vi "FIFO Core U128 - DRAM.vi"(0 "input data":cluster{"high":u64, "low":u64}, 1 "reset":bool, 2 "fifo memory":refnum<k21>, 3 "fifo depth":u8(ring)=10 items=["4"=2, "8"=3, "16"=4, "32"=5, "64"=6, "128"=7, "256"=8, "512"=9, "1024"=10, "2048"=11, "4096"=12, "8192"=13, "16384"=14, "32768"=15, "65536"=16, "131072"=17, "262144"=18, "524288"=19, "1048576"=20, "2097152"=21, "4194304"=22, "8388608"=23, "16777216"=24, "33554432"=25, "67108864"=26, "134217728"=27, "268435456"=28, "536870912"=29, "1073741824"=30, "2147483648"=31, "4294967296"=32], 5 "arbiter configuration":T2={"write grant time (clocks)"=100, "read grant time (clocks)"=100}, 9 "input valid":bool, 12 "ready for output":bool=TRUE) -> (4 "output data":cluster{"high":u64, "low":u64}, 6 "state":T1, 10 "output valid":bool, 14 "ready for input":bool)   [LabVIEW 2011, in "FIFO.lvlib"]
uses:
  <instrlib>/RF-RIO/FIFO/FIFO/FPGA/FIFO.lvlib
  <instrlib>/RF-RIO/FIFO/FIFO/FPGA/Public/FIFO State.ctl
  <instrlib>/RF-RIO/Memory/1.0.0/FPGA/Public/Write Data (128-Bit).ctl
  <instrlib>/RF-RIO/Memory/1.0.0/FPGA/Public/U128.ctl
  <instrlib>/FlexRIO/Libraries/Memory/FPGA/Interface/Read Request.ctl
  <instrlib>/RF-RIO/Memory/1.0.0/FPGA/Private/Process (DRAM 128-Bit).vi
  <instrlib>/FlexRIO/Libraries/Memory/FPGA/Memory.lvlib
  <instrlib>/RF-RIO/Memory/1.0.0/FPGA/niRFRIO Memory 1.0.0 FPGA.lvlib
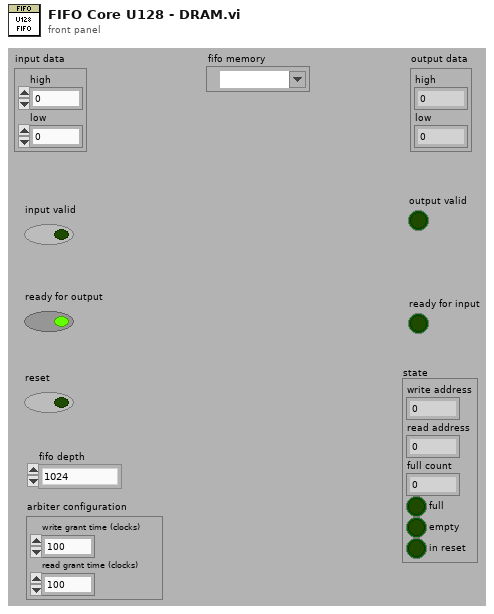
[diagram p1: front panel]
types:
  T1 = typedef "FIFO.lvlib/FIFO State.ctl" = cluster{"write address":u32, "read address":u32, "full count":u32, "full":bool, "empty":bool, "in reset":bool}
  T2 = cluster{"write grant time (clocks)":u16, "read grant time (clocks)":u16}
  T3 = typedef "Memory.lvlib/Read Request.ctl" = cluster{"address":u32, "valid":bool}
  T4 = typedef "FIFO.lvlib/niRFRIO Memory 1.0.0 FPGA.lvlib/Write Data (128-Bit).ctl" = cluster{"address":u32, "data":T5, "byte enables":u16, "valid":bool}
  T5 = typedef "FIFO.lvlib/niRFRIO Memory 1.0.0 FPGA.lvlib/U128.ctl" = cluster{"high":u64, "low":u64}
  T6 = typedef "FIFO.lvlib/FIFO State - 32-bit Address.ctl" = cluster{"write address":u32, "read address":u32, "full count":u32, "full":bool, "empty":bool}
  T7 = typedef "FIFO.lvlib/niRFRIO Memory 1.0.0 FPGA.lvlib/Retrieve Data (128-Bit).ctl" = cluster{"data":T5, "valid":bool}
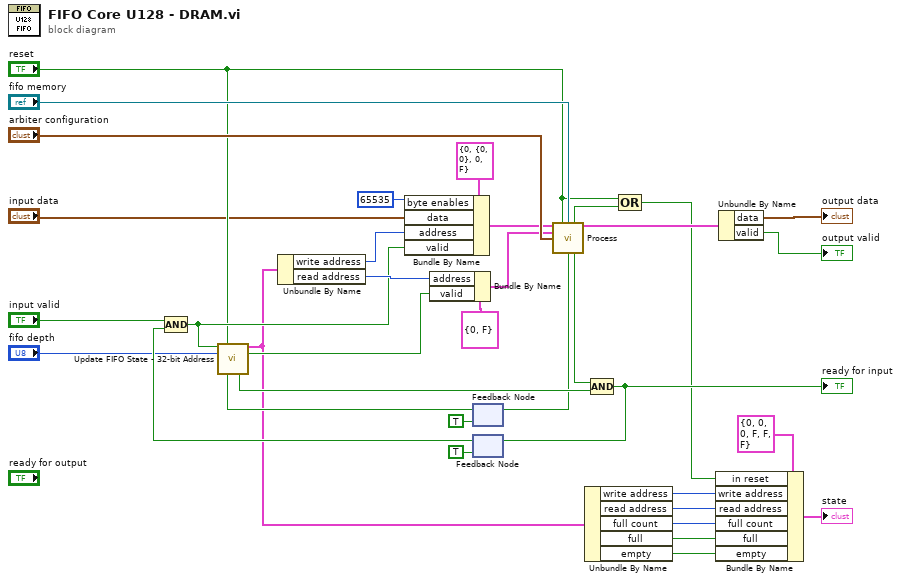
[diagram p0: block diagram]
diagram:
  n1 = feedback #1(TRUE ("ready for read request")) -> (w19:bool)
  n2 = feedback #2(TRUE) -> (w23:bool)
  n3 = Compound Arithmetic op=AND("input valid", w23) -> (w17:bool)
  n4 = call <instrlib>:"Update FIFO State - 32-bit Address.vi"("issue write"=w17, "reset"="reset", "fifo depth"="fifo depth", "ready for read request"=w19) -> ("state"=w6:T6, "issue read request"=w20:bool, "ready for write"=w22:bool)  [unwired: 9 in]
  n5 = Unbundle By Name(w6) -> ("write address"=w33:u32, "read address"=w29:u32)
  n6 = Bundle By Name(cluster=T4 {"address"=0, "data"={"high"=0, "low"=0}, "byte enables"=0, "valid"=FALSE} ("write data"), "byte enables"=u16 65535, "data"="input data", "address"=w33, "valid"=w17) -> (w3:T4)
  n7 = Bundle By Name(cluster=T3 {"address"=0, "valid"=FALSE} ("read request"), "address"=w29, "valid"=w20) -> (w30:T3)
  n8 = call-poly <instrlib>:"Process.vi"("write data"=w3, "reset"="reset", "memory"="fifo memory", "read request"=w30, "arbiter configuration"="arbiter configuration") -> ("in reset"=w9:bool, "retrieve data"=w27:T7, "ready for read request"=w21:bool, "ready for write"=w1:bool)  [unwired: 7 in]
  n9 = feedback-in #1(w21) -> ()
  n10 = Unbundle By Name(w6) -> ("write address"=w15:u32, "read address"=w14:u32, "full count"=w13:u32, "full"=w12:bool, "empty"=w11:bool)
  n11 = Compound Arithmetic op=AND(w1, w22) -> (w24:bool)
  "ready for input" <- w24
  n12 = feedback-in #2(w24) -> ()
  n13 = Compound Arithmetic op=OR("reset", w9) -> (w7:bool)
  n14 = Bundle By Name(cluster=T1 {"write address"=0, "read address"=0, "full count"=0, "full"=FALSE, "empty"=FALSE, "in reset"=FALSE} ("state"), "in reset"=w7, "write address"=w15, "read address"=w14, "full count"=w13, "full"=w12, "empty"=w11) -> (→"state":T1)
  n15 = Unbundle By Name(w27) -> ("data"=→"output data":T5, "valid"=→"output valid":bool)
